vi "MAVLink RX main.vi"() -> (0 "error out":errorcluster)   [LabVIEW 2014]
uses:
  Controls/MAVLink Packet.ctl
  Global Variables/Global Variables.vi
panel:
  out "Payload Length":u8
  out "Packet Sequence":u8 format="%x"
  out "System ID":u8
  out "Component ID":u8
  out "Message ID":u8
  out "Checksum":u16 format="%x"
  out "good crc":bool
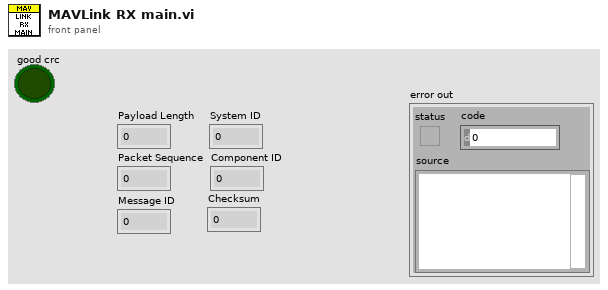
[diagram p1: front panel]
types:
  T1 = typedef "MAVLink Packet.ctl" = cluster{"Payload Length":u8, "Packet Sequence":u8, "System ID":u8, "Component ID":u8, "Message ID":u8, "Data":string, "Checksum":u16}
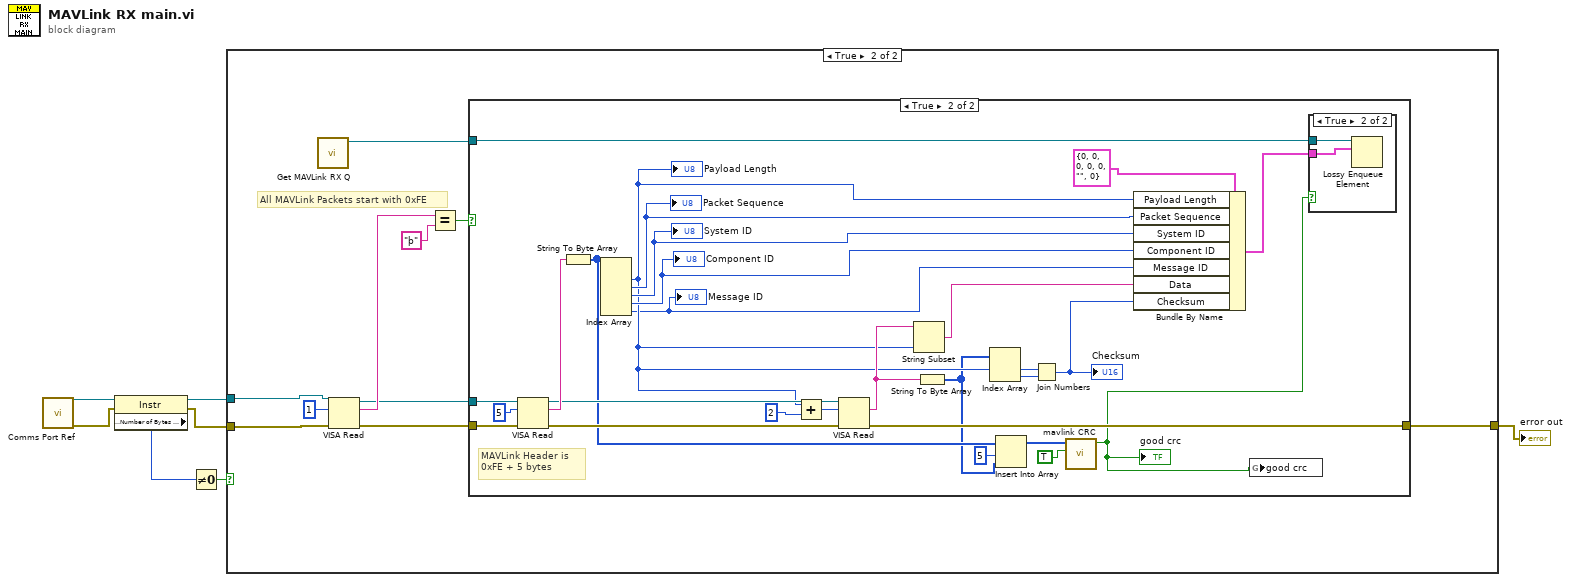
[diagram p0: block diagram]
diagram:
  n1 = call "Comms Port Ref.vi"() -> ("error out"=w3:errorcluster, "Comms Port Ref"=w4:refnum<visa-resource-name>)  [unwired: 10 in]
  n2 = property class="Instr"(reference=w4, error in=w3) -> (reference out=w6:refnum<visa-resource-name>, error out=w5:errorcluster, "Serial Settings:Number of Bytes at Serial Port"=w1:u32)
  n3 = Not Equal To 0?(x=w1) -> (x != 0?=w2:bool)
  n4 = case shown="True" w2 {
    tunnel: [w8 w18] -> w7
    tunnel: w5 -> [w8 w11]
    tunnel: w6 -> [_ w9]
    frame False {
    }
    frame True {
      # "All MAVLink Packets start with 0xFE"
      n5 = call "Get MAVLink RX Q.vi"() -> ("MAVLink RX Q"=w10:refnum<queue>)  [unwired: 10 in, 1 out]
      n6 = VISA Read(VISA resource name=w9, byte count=u32 1, error in (no error)=w11) -> (VISA resource name out=w13:refnum<visa-resource-name>, read buffer=w14:string, error out=w12:errorcluster)  [unwired: 1 out]
      n7 = Equal?(x=w14, y="þ") -> (x = y?=w16:bool)
      n8 = case shown="True" w16 {
        tunnel: w13 -> [_ w46]
        tunnel: w12 -> [w19 w45]
        tunnel: [w19 w40] -> w18
        tunnel: w10 -> [_ w30]
        frame False {
        }
        frame True {
          # "MAVLink Header is \n0xFE + 5 bytes"
          n9 = VISA Read(VISA resource name=w46, byte count=u32 5, error in (no error)=w45) -> (VISA resource name out=w43:refnum<visa-resource-name>, read buffer=w44:string, error out=w42:errorcluster)  [unwired: 1 out]
          n10 = String To Byte Array(string=w44) -> (unsigned byte array=w29:u8[])
          n11 = Index Array(array=w29) -> (element #1=w33:u8, element #2=w34:u8, element #3=w35:u8, element #4=w36:u8, element #5=w24:u8)  [unwired: 5 in]
          "Payload Length" <- w33
          "Packet Sequence" <- w34
          "System ID" <- w35
          "Component ID" <- w36
          "Message ID" <- w24
          n12 = Add(x=w33, y=u8 2) -> (x+y=w25:u8)
          n13 = VISA Read(VISA resource name=w43, byte count=w25, error in (no error)=w42) -> (read buffer=w39:string, error out=w40:errorcluster)  [unwired: 2 out]
          n14 = String Subset(string=w39, length (rest)=w33) -> (substring=w37:string)  [unwired: 1 in]
          n15 = String To Byte Array(string=w39) -> (unsigned byte array=w28:u8[])
          n16 = Index Array(array=w28, index #1=w33) -> (element #1=w32:u8, element #2=w31:u8)  [unwired: 1 in]
          n17 = Insert Into Array(array=w29, index=5, new element=w28) -> (w26:u8[])
          n18 = Join Numbers(hi=w32, lo=w31) -> ((hi.lo)=w38:u16)
          "Checksum" <- w38
          n19 = call "mavlink CRC.vi"("Check (T)/ Generate (F)"=TRUE ("Check / Generate"), "byte array input"=w26) -> ("good crc"=w20:bool)  [unwired: 8 in, 1 out]
          "good crc" <- w20
          n20 = Bundle By Name(cluster=T1 {"Payload Length"=0, "Packet Sequence"=0, "System ID"=0, "Component ID"=0, "Message ID"=0, "Data"="", "Checksum"=0} ("MAVLink Packet"), "Payload Length"=w33, "Packet Sequence"=w34, "System ID"=w35, "Component ID"=w36, "Message ID"=w24, "Data"=w37, "Checksum"=w38) -> (w23:T1)
          n21 = global write "Global Variables.vi" "good crc"(w20) -> ()
          n22 = case shown="True" w20 {
            tunnel: w23 -> [_ w49]
            tunnel: w30 -> [_ w48]
            frame False {
            }
            frame True {
              n23 = Lossy Enqueue Element(queue=w48, element=w49) -> ()  [unwired: 1 in, 4 out]
            }
          }
        }
      }
    }
  }
  "error out" <- w7
